vi "Untitled 1.vi"() -> ()   [LabVIEW 2016]
panel:
  in  "Slide":dbl(slide) scale=-20.0..30.0
  in  "Ring":u16(ring)
  in  "OK Button":bool
  out "Boolean":bool
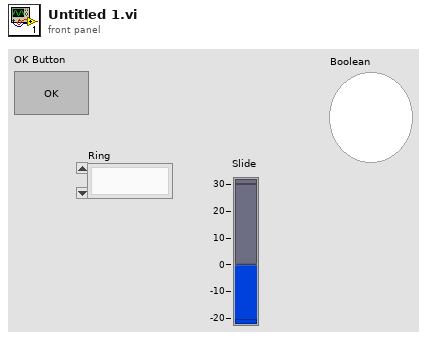
[diagram p1: front panel]
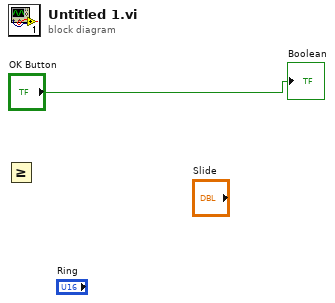
[diagram p0: block diagram]
diagram:
  n1 = Greater Or Equal?() -> ()  [unwired: 2 in, 1 out]
  "Boolean" <- "OK Button"
